vi "FRCts20_Backend_API_Division.vi"(8 "error in (no error)":errorcluster, 10 "Command":T1="GetDivision", 11 "Division In":T2) -> (0 "error out":errorcluster, 2 "Status":string, 3 "Division Out":T2)   [LabVIEW 2014, in "FRCts20_Backend_API.lvlib"]
doc: "This API call is in charge of returning all information about a division, including teams. It also handles any command which returns just team numbers, such as all teams in existence or all teams in a given competition."
uses:
  FRCts20_Backend_API.lvlib
  FRCts20_Backend_API_Division.ctl
  FRCts20_Backend_API_SW.ctl
  FRCts20_Backend_API_Status.ctl
  FRCts20_Backend_API_Command_Division.ctl
  FRCts20_Backend_FGVOperation.ctl
  FRCts20_Backend_Engine.lvlib
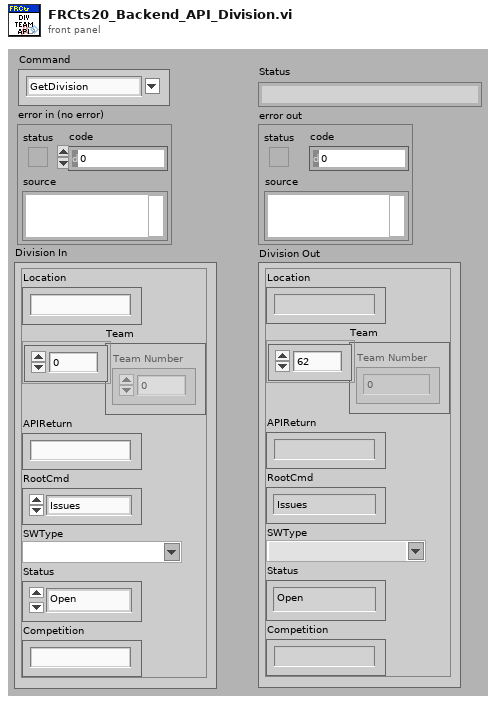
[diagram p1: front panel]
types:
  T1 = typedef "FRCts20_Backend_API.lvlib/FRCts20_Backend_API_Command_Division.ctl" = string
  T2 = typedef "FRCts20_Backend_API.lvlib/FRCts20_Backend_API_Division.ctl" = cluster{"Location":string, "Team":u32[], "APIReturn":string, "RootCmd":enum16{"Issues", "Software", "All"}, "SWType":T3, "Status":T4, "Competition":string}
  T3 = typedef "FRCts20_Backend_API.lvlib/FRCts20_Backend_API_SW.ctl" = string
  T4 = typedef "FRCts20_Backend_API.lvlib/FRCts20_Backend_API_Status.ctl" = enum16{"Open", "In Work", "Closed"}
  T5 = typedef "FRCts20_Backend_Engine.lvlib/FRCts20_Backend_FGVOperation.ctl" = enum16{"Initialize", "EnqueueMessage", "EnqueueDataReturn", "FlushMessage", "FlushDataReturn"}
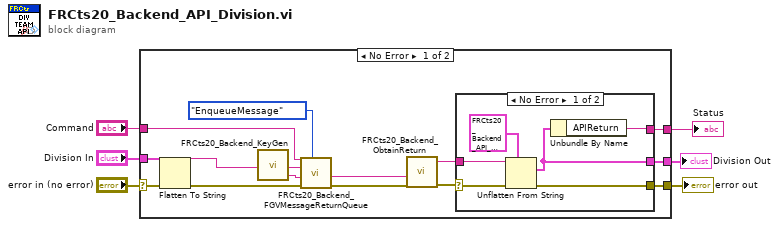
[diagram p0: block diagram]
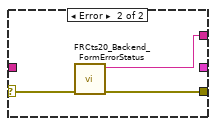
[diagram p2: hidden frame]
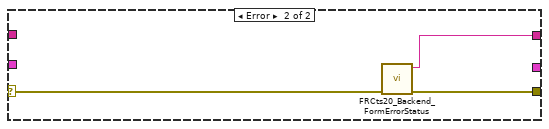
[diagram p3: hidden frame]
diagram:
  n1 = case shown="No Error" "error in (no error)" {
    selector: "error in (no error)" -> [w19 w31]
    tunnel: [w9 w32] -> w5
    tunnel: [w7 w30] -> w4
    tunnel: "Command" -> [w13 _]
    tunnel: "Division In" -> [w12 _]
    tunnel: [w8 _] -> w1
    frame No Error {
      n2 = Flatten To String(anything=w12, error in (no error)=w19) -> (data string=w20:string, error out=w18:errorcluster)  [unwired: 2 in, 1 out]
      n3 = call "FRCts20_Backend_KeyGen.vi"() -> ("Keygen"=w17:string)  [unwired: 27 in]
      n4 = call "FRCts20_Backend_FGVMessageReturnQueue.vi"("Operation"=FRCts20_Backend_FGVOperation."EnqueueMessage", "error in (no error)"=w18, "Key"=w17, "Message Value"=w20, "Message Name"=w13) -> ("error out"=w15:errorcluster, "Key (Duplicate)"=w14:string)  [unwired: 5 in]
      n5 = call "FRCts20_Backend_ObtainReturn.vi"("error in (no error)"=w15, "Key"=w14) -> ("error out"=w11:errorcluster, "Message Value"=w10:string)  [unwired: 8 in]
      n6 = case shown="No Error" w11 {
        selector: w11 -> [w25 w29]
        tunnel: [w26 w28] -> w9
        tunnel: [w24 _] -> w8
        tunnel: [w23 w27] -> w7
        tunnel: w10 -> [w22 _]
        frame No Error {
          n7 = Unflatten From String(type=T2 {"Location"="", "Team"=[], "APIReturn"="", "RootCmd"=enum."Issues", "SWType"="", "Status"=enum."Open", "Competition"=""} ("Division"), binary string=w22, error in (no error)=w25) -> (value=w24:T2, error out=w26:errorcluster)  [unwired: 2 in, 1 out]
          n8 = Unbundle By Name(w24) -> ("APIReturn"=w23:string)
        }
        frame Error {
          n9 = call "FRCts20_Backend_FormErrorStatus.vi"("error in (no error)"=w29) -> ("error out"=w28:errorcluster, "String"=w27:string)  [unwired: 9 in]
        }
      }
    }
    frame Error {
      n10 = call "FRCts20_Backend_FormErrorStatus.vi"("error in (no error)"=w31) -> ("error out"=w32:errorcluster, "String"=w30:string)  [unwired: 9 in]
    }
  }
  "error out" <- w5
  "Status" <- w4
  "Division Out" <- w1
